vi "get latest tdms path.vi"(11 "scans path":path) -> (3 "latest tdms":path)   [LabVIEW 2020]
uses:
  <userlib>/_OpenG.lib/array/array.llb/Sort 1D Array (I32)__ogtk.vi
panel:
  out "latest scan path":path
  out "element":string
  out "Array":i32[](array[numeric])
  out "folder names":string[](array[string])
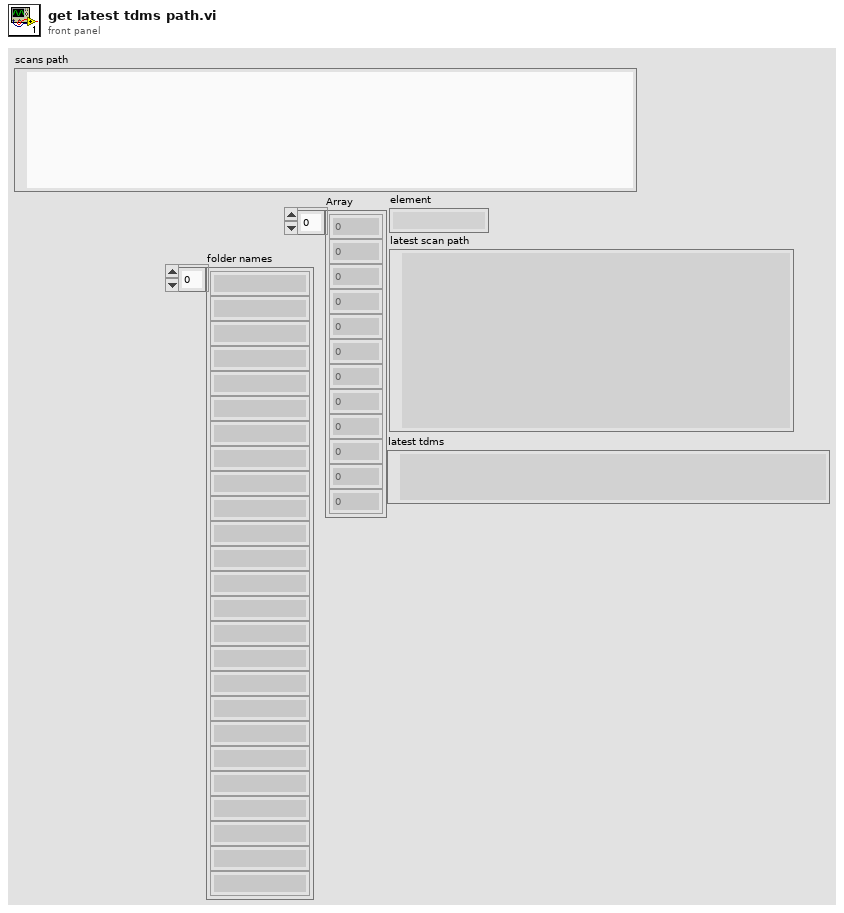
[diagram p1: front panel]
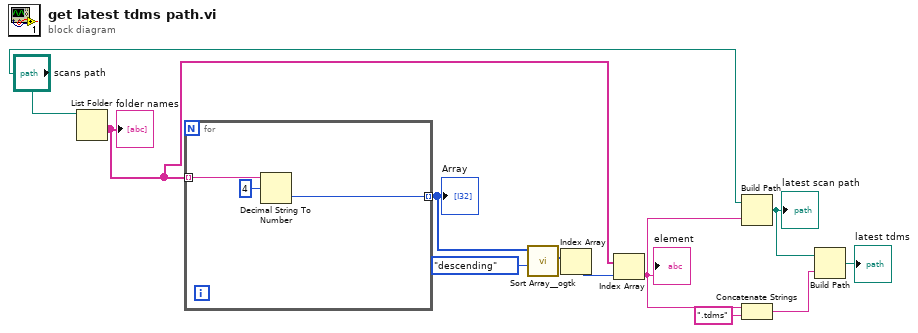
[diagram p0: block diagram]
diagram:
  n1 = List Folder(path="scans path") -> (folder names=w9:string[])  [unwired: 3 in, 3 out]
  "folder names" <- w9
  n2 = for {
    tunnel: w9 -> [w14] mode=indexing
    tunnel: [w13] -> w11 mode=indexing
    n3 = Decimal String To Number(string=w14, offset=4) -> (number=w13:i32)  [unwired: 1 in, 1 out]
  }
  "Array" <- w11
  n4 = call-poly <userlib>:"Sort Array__ogtk.vi"("Order"=enum16{"ascending", "descending"}."descending", "Array in"=w11) -> ("Sorted Pointers"=w8:i32[])  [unwired: 8 in, 1 out]
  n5 = Index Array(array=w8) -> (element=w7:i32)  [unwired: 1 in]
  n6 = Index Array(array=w9, index=w7) -> (element=w5:string)
  "element" <- w5
  n7 = Build Path(base path="scans path", name or relative path=w5) -> (appended path=w3:path)
  "latest scan path" <- w3
  n8 = Concatenate Strings(w5, ".tdms" ("string")) -> (w2:string)
  n9 = Build Path(base path=w3, name or relative path=w2) -> (appended path=→"latest tdms":path)
